vi "UTILITY Modbus 32bit Number Combine.vi"(10 "Swap Words":bool=TRUE, 11 "Holding Registers":u16[](array[numeric]) format="%.0x") -> (2 "word swapped":u32 format="%.0x", 3 "Data":sgl)   [LabVIEW 2019]
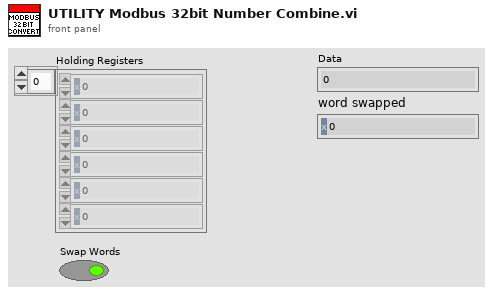
[diagram p1: front panel]
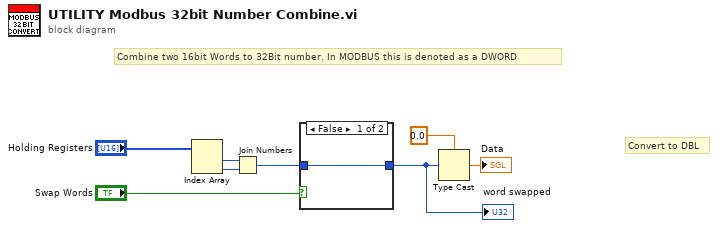
[diagram p0: block diagram]
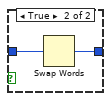
[diagram p2: hidden frame]
diagram:
  # "Convert to DBL"
  # "Combine two 16bit Words to 32Bit number. In MODBUS this is denoted as a DWORD"
  n1 = Index Array(array="Holding Registers") -> (element #1=w3:u16, element #2=w5:u16)  [unwired: 2 in]
  n2 = Join Numbers(hi=w3, lo=w5) -> ((hi.lo)=w2:u32)
  n3 = case shown="False" "Swap Words" {
    tunnel: [w9 w11] -> w4
    tunnel: w2 -> [w9 w10]
    frame False {
    }
    frame True {
      n4 = Swap Words(1:w10) -> (0:w11:u32)
    }
  }
  "word swapped" <- w4
  n5 = Type Cast(type=sgl 0.0, x=w4) -> (*(type *) &x=→"Data":sgl)
